vi "WriteToCSV.vi"(11 "Input":string[][](array[string])) -> ()   [LabVIEW 2020, in "WritingDataFile.lvlib"]
uses:
  WritingDataFile/WritingDataFile.lvlib
  <vilib>/Utility/file.llb/Write Delimited Spreadsheet (string).vi
panel:
  out "Flue Gas Temperature Top":string[](array[string])
  out "Millivoltage Output Pilot (mV)":string[](array[string])
  out "Flue Gas Baffle Temperature Bottom":string[](array[string])
  out "Output array":string[][](array[string])
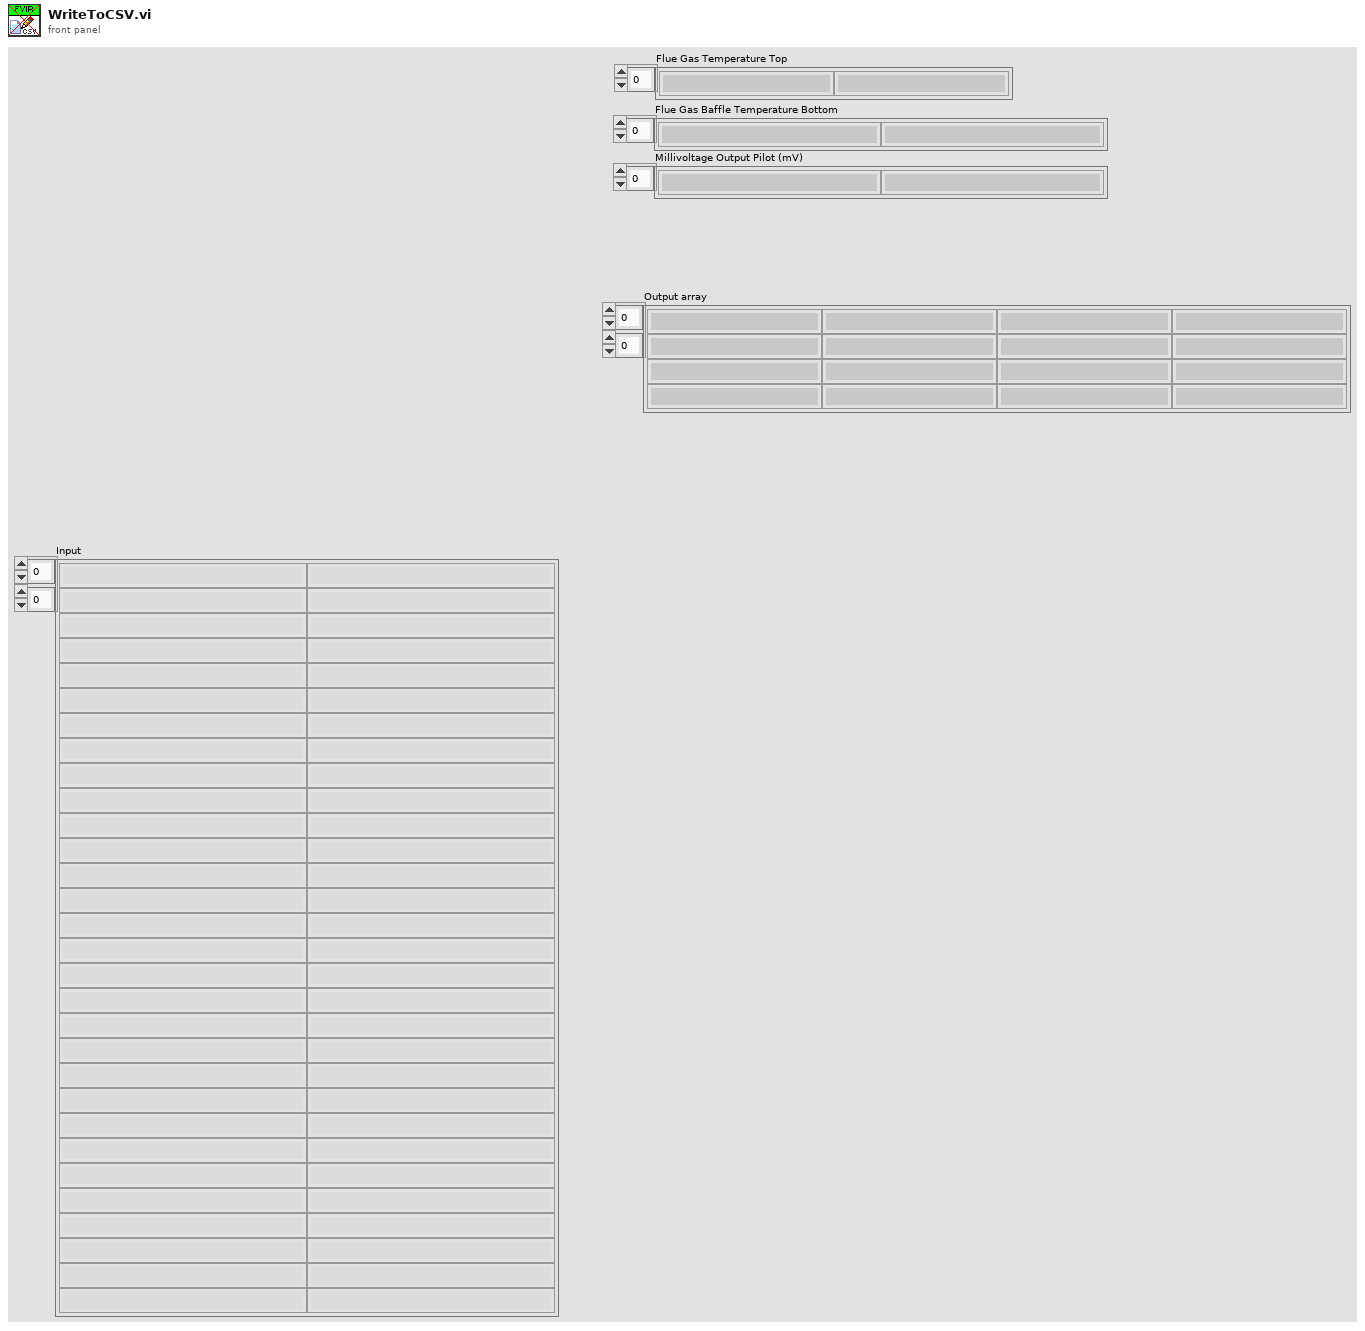
[diagram p1: front panel]
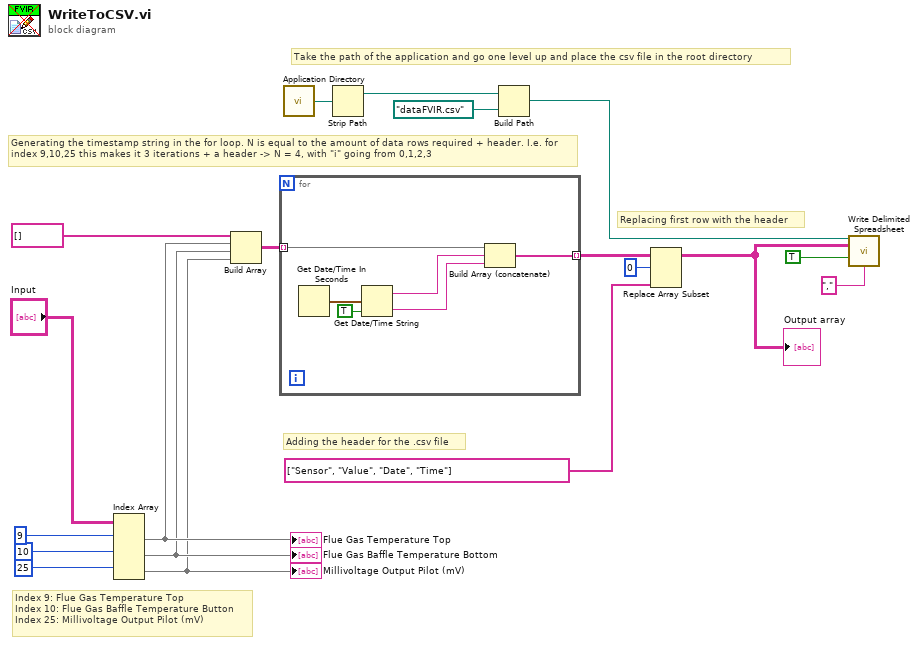
[diagram p0: block diagram]
diagram:
  # "Replacing first row with the header"
  # "Generating the timestamp string in the for loop. N is equal to the amount of data rows required + header. I.e. for index 9,10,25 this makes it 3 iterations + a header -> N = 4, with \"i\" going from 0,1,2,3"
  # "Index 9: Flue Gas Temperature Top\nIndex 10: Flue Gas Baffle Temperature Button\nIndex 25: Millivoltage Output Pilot (mV)"
  # "Adding the header for the .csv file"
  # "Take the path of the application and go one level up and place the csv file in the root directory"
  n1 = Index Array(array="Input", index (row) #1=9 ("index (row)"), index (row) #2=10 ("index (row)"), index (row) #3=25 ("index (row)")) -> (element #1=w6:string[], element #2=w5:string[], element #3=w4:string[])  [unwired: 3 in]
  "Flue Gas Baffle Temperature Bottom" <- w5
  "Millivoltage Output Pilot (mV)" <- w4
  "Flue Gas Temperature Top" <- w6
  n2 = Build Array(string[] [] ("element"), w6, w5, w4) -> (w3:string[][])
  n3 = for {
    tunnel: w3 -> [w25] mode=indexing
    tunnel: [w20] -> w19 mode=indexing
    n4 = Get Date/Time In Seconds() -> (seconds since 1Jan1904=w24:timestamp)
    n5 = Get Date/Time String(seconds (now)=w24, want seconds? (F)=TRUE) -> (date string=w22:string, time string=w21:string)  [unwired: 1 in]
    n6 = Build Array (concatenate)(w25, w22, w21) -> (w20:string[])
  }
  n7 = call <vilib>:"Application Directory.vi"() -> ("Application Directory"=w16:path)
  n8 = Strip Path(path=w16) -> (stripped path=w14:path)  [unwired: 1 out]
  n9 = Build Path(base path=w14, name or relative path=path "dataFVIR.csv") -> (appended path=w12:path)
  n10 = Replace Array Subset(array=w19, new element=string[] ["Sensor", "Value", "Date", "Time"] ("new element/subarray"), index (row)=0) -> (w1:string[][])  [unwired: 1 in]
  "Output array" <- w1
  n11 = call-poly <vilib>:"Write Delimited Spreadsheet.vi"("file path (dialog if empty)"=w12, "2D data"=w1, "append to file? (new file:F)"=TRUE, "delimiter (\\t)"="," ("delimiter (\\t)")) -> ()  [unwired: 10 in, 2 out]
